vi "fita2.vi"() -> ()   [LabVIEW 2014]
uses:
  <vilib>/Analysis/5stat.llb/RMS (DBL).vi
  <vilib>/DAQmx/create/channels.llb/DAQmx Create Channel (AI-Voltage-Basic).vi
  <vilib>/DAQmx/configure/timing.llb/DAQmx Timing (Sample Clock).vi
  <vilib>/DAQmx/read.llb/DAQmx Read (Analog 1D Wfm NChan NSamp).vi
  <vilib>/Waveform/WDTOps.llb/WDT Index Channel DBL.vi
  <vilib>/Utility/file.llb/Write To Spreadsheet File (string).vi
  <vilib>/Analysis/NI_AALPro.lvlib
panel:
  out "CH4":dbl
  out "CH3":dbl
  out "CH2":dbl
  out "CH1":dbl
  out "MIN CH4":bool
  out "MIN CH2":bool
  out "MIN CH1":bool
  out "MIN CH3":bool
  out "MAX CH4":bool
  out "MAX CH3":bool
  out "MAX CH2":bool
  out "MAX CH1":bool
  in  "Temp Max CH2":dbl
  in  "Temp Min CH1":dbl
  in  "Temp Min CH2":dbl
  in  "Temp Max CH3":dbl
  in  "Temp Min CH3":dbl
  in  "Temp Max CH4":dbl
  in  "Temp Min CH4":dbl
  in  "Temp Max CH1":dbl
  in  "Start":bool
  in  "stop":bool
  out "Waveform Chart":T1(graph)
  out "Canals seleccionats":dbl
  in  "Durada adquisicio":dbl
  in  "Temps entre adquisicio":dbl
  in  "Numero de mostres per fer mitja":u32
  in  "Nombre de Canals":string(combo)
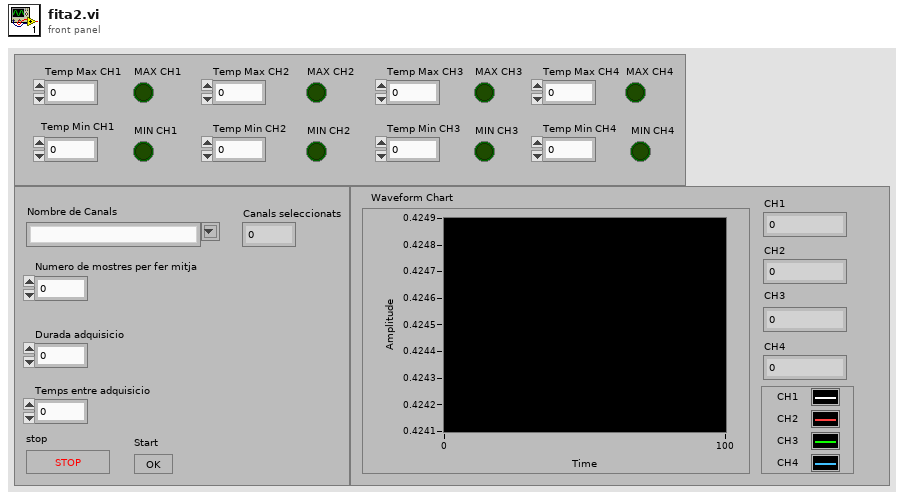
[diagram p1: front panel]
types:
  T1 = cluster{"rms value":dbl, "rms value":dbl, "rms value":dbl, "rms value":dbl}
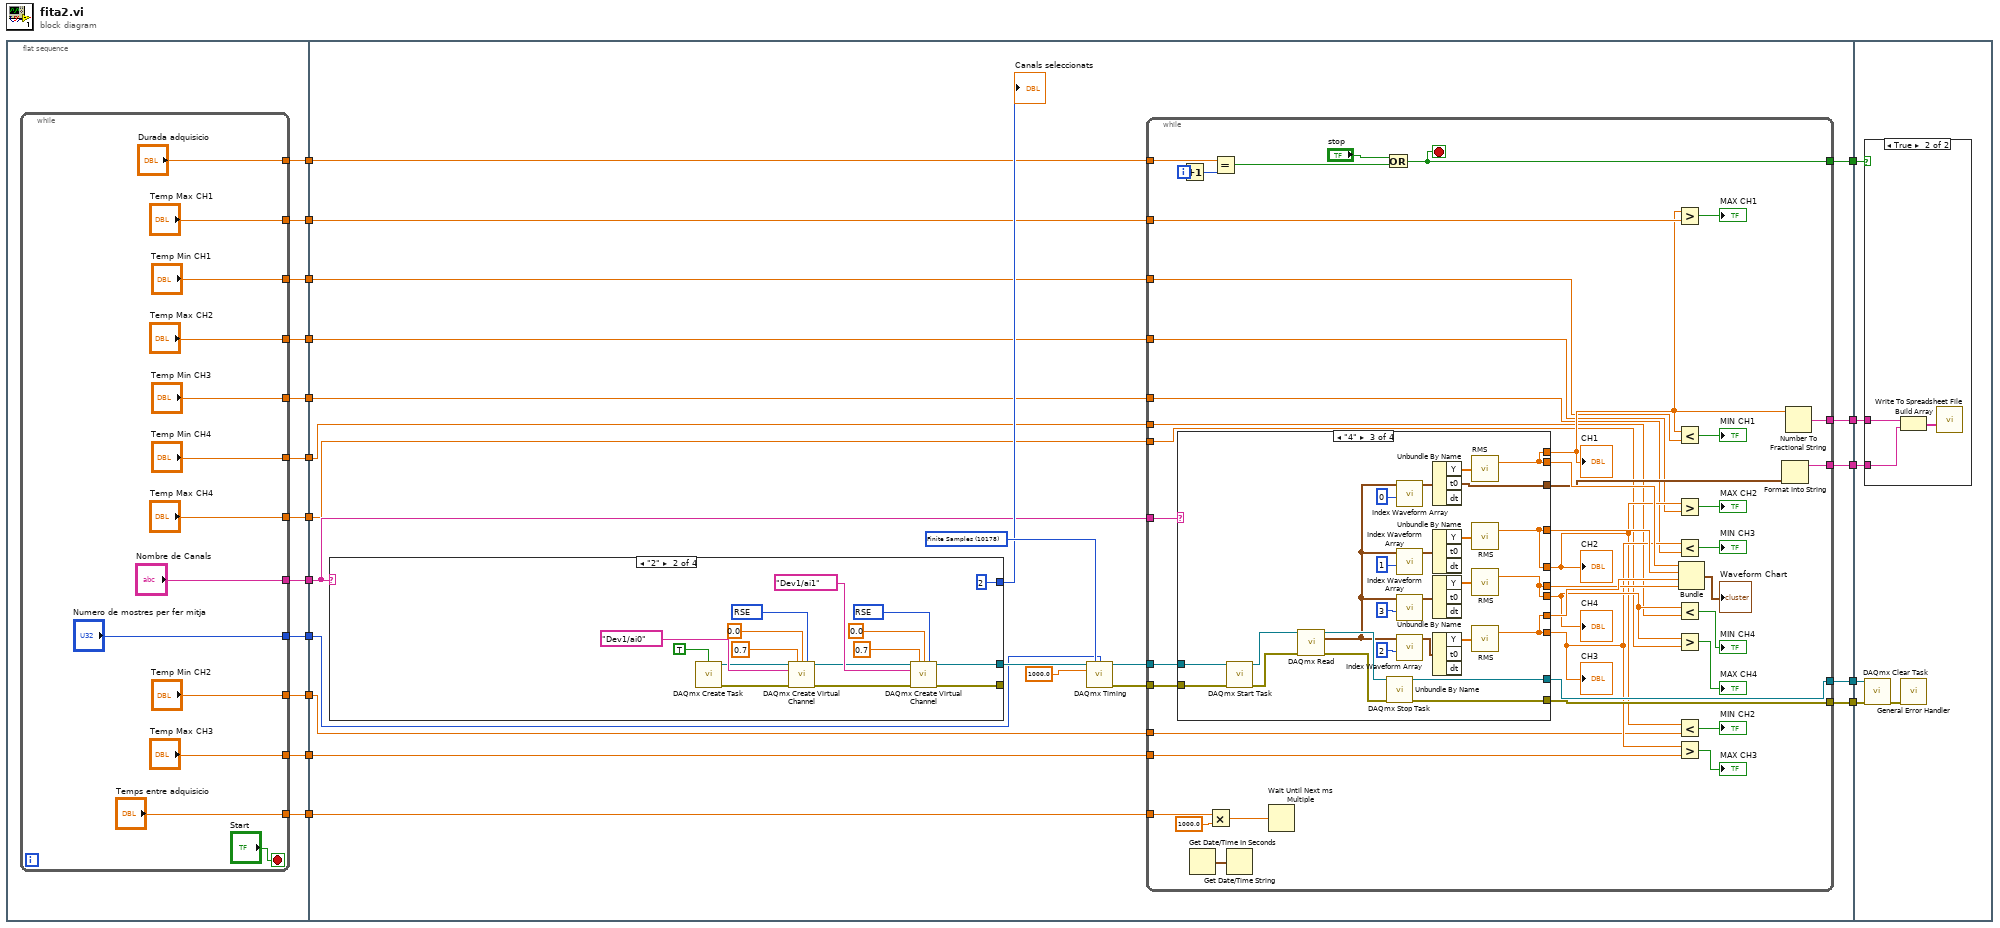
[diagram p0: block diagram]
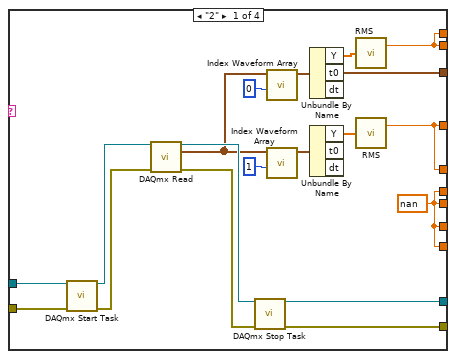
[diagram p2: hidden frame]
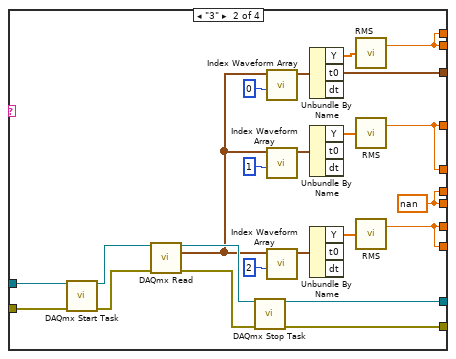
[diagram p3: hidden frame]
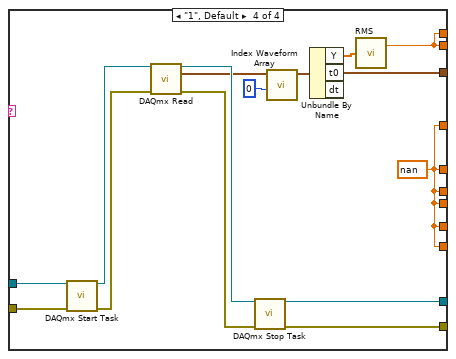
[diagram p4: hidden frame]
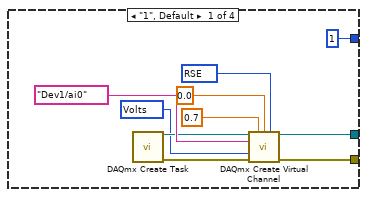
[diagram p5: hidden frame]
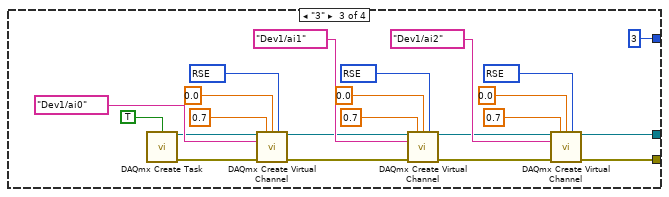
[diagram p6: hidden frame]
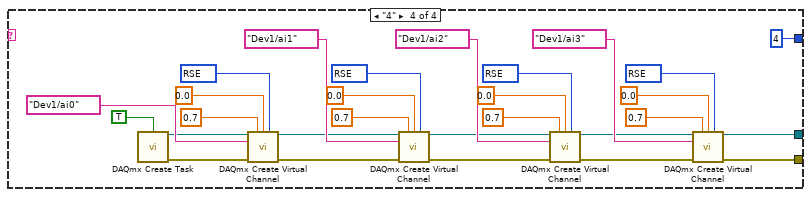
[diagram p7: hidden frame]
diagram:
  n1 = flat-sequence {
    tunnel: [w29] -> w17
    tunnel: [w28] -> w16
    tunnel: [w27] -> w15
    tunnel: [w26] -> w14
    tunnel: [w25] -> w8
    tunnel: [w24] -> w7
    tunnel: [w23] -> w6
    tunnel: [w22] -> w5
    tunnel: [w21] -> w4
    tunnel: [w20] -> w3
    tunnel: [w19] -> w2
    tunnel: [w18] -> w1
    tunnel: w17 -> [w59]
    tunnel: w16 -> [w58]
    tunnel: w15 -> [w57]
    tunnel: w14 -> [w56]
    tunnel: [w55] -> w13
    tunnel: [w54] -> w12
    tunnel: [w53] -> w11
    tunnel: [w52] -> w10
    tunnel: [w51] -> w9
    tunnel: w8 -> [w50]
    tunnel: w7 -> [w49]
    tunnel: w6 -> [w48]
    tunnel: w5 -> [w47]
    tunnel: w4 -> [w46]
    tunnel: w3 -> [w45]
    tunnel: w2 -> [w44]
    tunnel: w1 -> [w43]
    tunnel: w13 -> [w272]
    tunnel: w12 -> [w271]
    tunnel: w11 -> [w270]
    tunnel: w10 -> [w269]
    tunnel: w9 -> [w268]
    frame #0 {
      n2 = while {
        tunnel: ["Nombre de Canals"] -> w29
        tunnel: ["Durada adquisicio"] -> w28
        tunnel: ["Temps entre adquisicio"] -> w27
        tunnel: ["Numero de mostres per fer mitja"] -> w26
        tunnel: ["Temp Max CH1"] -> w25
        tunnel: ["Temp Min CH1"] -> w24
        tunnel: ["Temp Max CH3"] -> w23
        tunnel: ["Temp Max CH2"] -> w22
        tunnel: ["Temp Max CH4"] -> w21
        tunnel: ["Temp Min CH3"] -> w20
        tunnel: ["Temp Min CH2"] -> w19
        tunnel: ["Temp Min CH4"] -> w18
        stop <- "Start" stop-if-true
      }
    }
    frame #1 {
      w64 = 10178 items=["Finite Samples"=10178, "Continuous Samples"=10123, "Hardware Timed Single Point"=12522] ("sample mode")
      n3 = case shown="\"2\"" w59 {
        tunnel: [w195 w204 w220 w242] -> w65
        tunnel: [w194 w203 w219 w241] -> _
        tunnel: [1 2 3 4] -> w63
        frame "1", Default {
          w192 = 10348 items=["Volts"=10348, "From Custom Scale"=10065] ("units")
          w198 = 10083 items=["default"=-1, "RSE"=10083, "NRSE"=10078, "Differential"=10106, "Pseudodifferential"=12529] ("input terminal configuration")
          n4 = call <vilib>:"DAQmx Create Task.vi"() -> ("task out"=w196:refnum<k21>, "error out"=w197:errorcluster)  [unwired: 14 in]
          n5 = call-poly <vilib>:"DAQmx Create Virtual Channel.vi"("task in"=w196, "maximum value"=0.7, "minimum value"=0.0, "input terminal configuration"=w198, "physical channels"=tag "Dev1/ai0", "units"=w192, "error in"=w197) -> ("task out"=w195:refnum<k21>, "error out"=w194:errorcluster)  [unwired: 7 in]
        }
        frame "2" {
          w207 = 10083 items=["default"=-1, "RSE"=10083, "NRSE"=10078, "Differential"=10106, "Pseudodifferential"=12529] ("input terminal configuration")
          w214 = 10083 items=["default"=-1, "RSE"=10083, "NRSE"=10078, "Differential"=10106, "Pseudodifferential"=12529] ("input terminal configuration")
          n6 = call <vilib>:"DAQmx Create Task.vi"("auto cleanup"=TRUE) -> ("task out"=w212:refnum<k21>, "error out"=w213:errorcluster)  [unwired: 13 in]
          n7 = call-poly <vilib>:"DAQmx Create Virtual Channel.vi"("task in"=w212, "maximum value"=0.7, "minimum value"=0.0, "input terminal configuration"=w214, "physical channels"=tag "Dev1/ai0", "error in"=w213) -> ("task out"=w206:refnum<k21>, "error out"=w205:errorcluster)  [unwired: 8 in]
          n8 = call-poly <vilib>:"DAQmx Create Virtual Channel.vi"("task in"=w206, "maximum value"=0.7, "minimum value"=0.0, "input terminal configuration"=w207, "physical channels"=tag "Dev1/ai1", "error in"=w205) -> ("task out"=w204:refnum<k21>, "error out"=w203:errorcluster)  [unwired: 8 in]
        }
        frame "3" {
          w223 = 10083 items=["default"=-1, "RSE"=10083, "NRSE"=10078, "Differential"=10106, "Pseudodifferential"=12529] ("input terminal configuration")
          w229 = 10083 items=["default"=-1, "RSE"=10083, "NRSE"=10078, "Differential"=10106, "Pseudodifferential"=12529] ("input terminal configuration")
          w236 = 10083 items=["default"=-1, "RSE"=10083, "NRSE"=10078, "Differential"=10106, "Pseudodifferential"=12529] ("input terminal configuration")
          n9 = call <vilib>:"DAQmx Create Task.vi"("auto cleanup"=TRUE) -> ("task out"=w234:refnum<k21>, "error out"=w235:errorcluster)  [unwired: 13 in]
          n10 = call-poly <vilib>:"DAQmx Create Virtual Channel.vi"("task in"=w234, "maximum value"=0.7, "minimum value"=0.0, "input terminal configuration"=w236, "physical channels"=tag "Dev1/ai0", "error in"=w235) -> ("task out"=w228:refnum<k21>, "error out"=w227:errorcluster)  [unwired: 8 in]
          n11 = call-poly <vilib>:"DAQmx Create Virtual Channel.vi"("task in"=w228, "maximum value"=0.7, "minimum value"=0.0, "input terminal configuration"=w229, "physical channels"=tag "Dev1/ai1", "error in"=w227) -> ("task out"=w222:refnum<k21>, "error out"=w221:errorcluster)  [unwired: 8 in]
          n12 = call-poly <vilib>:"DAQmx Create Virtual Channel.vi"("task in"=w222, "maximum value"=0.7, "minimum value"=0.0, "input terminal configuration"=w223, "physical channels"=tag "Dev1/ai2", "error in"=w221) -> ("task out"=w220:refnum<k21>, "error out"=w219:errorcluster)  [unwired: 8 in]
        }
        frame "4" {
          w245 = 10083 items=["default"=-1, "RSE"=10083, "NRSE"=10078, "Differential"=10106, "Pseudodifferential"=12529] ("input terminal configuration")
          w251 = 10083 items=["default"=-1, "RSE"=10083, "NRSE"=10078, "Differential"=10106, "Pseudodifferential"=12529] ("input terminal configuration")
          w257 = 10083 items=["default"=-1, "RSE"=10083, "NRSE"=10078, "Differential"=10106, "Pseudodifferential"=12529] ("input terminal configuration")
          w264 = 10083 items=["default"=-1, "RSE"=10083, "NRSE"=10078, "Differential"=10106, "Pseudodifferential"=12529] ("input terminal configuration")
          n13 = call <vilib>:"DAQmx Create Task.vi"("auto cleanup"=TRUE) -> ("task out"=w262:refnum<k21>, "error out"=w263:errorcluster)  [unwired: 13 in]
          n14 = call-poly <vilib>:"DAQmx Create Virtual Channel.vi"("task in"=w262, "maximum value"=0.7, "minimum value"=0.0, "input terminal configuration"=w264, "physical channels"=tag "Dev1/ai0", "error in"=w263) -> ("task out"=w256:refnum<k21>, "error out"=w255:errorcluster)  [unwired: 8 in]
          n15 = call-poly <vilib>:"DAQmx Create Virtual Channel.vi"("task in"=w256, "maximum value"=0.7, "minimum value"=0.0, "input terminal configuration"=w257, "physical channels"=tag "Dev1/ai1", "error in"=w255) -> ("task out"=w250:refnum<k21>, "error out"=w249:errorcluster)  [unwired: 8 in]
          n16 = call-poly <vilib>:"DAQmx Create Virtual Channel.vi"("task in"=w250, "maximum value"=0.7, "minimum value"=0.0, "input terminal configuration"=w251, "physical channels"=tag "Dev1/ai2", "error in"=w249) -> ("task out"=w244:refnum<k21>, "error out"=w243:errorcluster)  [unwired: 8 in]
          n17 = call-poly <vilib>:"DAQmx Create Virtual Channel.vi"("task in"=w244, "maximum value"=0.7, "minimum value"=0.0, "input terminal configuration"=w245, "physical channels"=tag "Dev1/ai3", "error in"=w243) -> ("task out"=w242:refnum<k21>, "error out"=w241:errorcluster)  [unwired: 8 in]
        }
      }
      "Canals seleccionats" <- w63
      n18 = call-poly <vilib>:"DAQmx Timing.vi"("task/channels in"=w65, "sample mode"=w64, "samples per channel"=w56, "rate"=1000.0) -> ("task out"=w61:refnum<k21>, "error out"=w60:errorcluster)  [unwired: 10 in]
      n19 = while {
        tunnel: w57 -> [w106]
        tunnel: w59 -> [w105]
        tunnel: w61 -> [w104]
        tunnel: w60 -> [w103]
        tunnel: [w102] -> w55
        tunnel: [w101] -> w54
        tunnel: w58 -> [w92]
        tunnel: [w91] -> w53
        tunnel: [w87] -> w52
        tunnel: [w88] -> w51
        tunnel: w50 -> [w86]
        tunnel: w49 -> [w82]
        tunnel: w48 -> [w71]
        tunnel: w47 -> [w70]
        tunnel: w46 -> [w69]
        tunnel: w45 -> [w68]
        tunnel: w44 -> [w67]
        tunnel: w43 -> [w66]
        i -> [w98]
        stop <- w91 stop-if-true
        n20 = case shown="\"4\"" w105 {
          tunnel: w104 -> [w116 w136 w159 w183]
          tunnel: w103 -> [w115 w135 w158 w182]
          tunnel: [w114 w134 w157 w181] -> w102
          tunnel: [w113 w133 w156 w180] -> w101
          tunnel: [w112 w131 w155 w179] -> w96
          tunnel: [w111 w130 w154 w178] -> w95
          tunnel: [w110 w132 w153 w178] -> w93
          tunnel: [w110 w129 w152 w178] -> w75
          tunnel: [w112 w131 w155 w179] -> w85
          tunnel: [w111 w130 w154 w178] -> w72
          tunnel: [w110 w132 w153 w178] -> w73
          tunnel: [w110 w129 w152 w178] -> w74
          tunnel: [w109 w128 w151 w177] -> w89
          frame "2" {
            w110 = nan ("rms value")
            n21 = call <vilib>:"DAQmx Start Task.vi"("task/channels in"=w116, "error in"=w115) -> ("task out"=w127:refnum<k21>, "error out"=w126:errorcluster)  [unwired: 12 in]
            n22 = call-poly <vilib>:"DAQmx Read.vi"("task/channels in"=w127, "error in"=w126) -> ("task out"=w124:refnum<k21>, "data"=w117:waveform(dbl)[], "error out"=w125:errorcluster)  [unwired: 11 in]
            n23 = call <vilib>:"DAQmx Stop Task.vi"("task/channels in"=w124, "error in"=w125) -> ("task out"=w114:refnum<k21>, "error out"=w113:errorcluster)  [unwired: 12 in]
            n24 = call-poly <vilib>:"Index Waveform Array.vi"("index"=0, "waveform array"=w117) -> ("waveform"=w119:waveform(dbl))  [unwired: 8 in, 1 out]
            n25 = call-poly <vilib>:"Index Waveform Array.vi"("index"=1, "waveform array"=w117) -> ("waveform"=w122:waveform(dbl))  [unwired: 8 in, 1 out]
            n26 = Unbundle By Name(w119) -> ("Y"=w118:dbl[], "t0"=w109:timestamp)  [unwired: 1 out]
            n27 = Unbundle By Name(w122) -> ("Y"=w121:dbl[])  [unwired: 2 out]
            n28 = call-poly <vilib>:"RMS.vi"("X"=w118) -> ("rms value"=w112:dbl)  [unwired: 1 out]
            n29 = call-poly <vilib>:"RMS.vi"("X"=w121) -> ("rms value"=w111:dbl)  [unwired: 1 out]
          }
          frame "3" {
            w129 = nan ("rms value")
            n30 = call <vilib>:"DAQmx Start Task.vi"("task/channels in"=w136, "error in"=w135) -> ("task out"=w150:refnum<k21>, "error out"=w149:errorcluster)  [unwired: 12 in]
            n31 = call-poly <vilib>:"DAQmx Read.vi"("task/channels in"=w150, "error in"=w149) -> ("task out"=w147:refnum<k21>, "data"=w137:waveform(dbl)[], "error out"=w148:errorcluster)  [unwired: 11 in]
            n32 = call <vilib>:"DAQmx Stop Task.vi"("task/channels in"=w147, "error in"=w148) -> ("task out"=w134:refnum<k21>, "error out"=w133:errorcluster)  [unwired: 12 in]
            n33 = call-poly <vilib>:"Index Waveform Array.vi"("index"=0, "waveform array"=w137) -> ("waveform"=w142:waveform(dbl))  [unwired: 8 in, 1 out]
            n34 = call-poly <vilib>:"Index Waveform Array.vi"("index"=1, "waveform array"=w137) -> ("waveform"=w139:waveform(dbl))  [unwired: 8 in, 1 out]
            n35 = call-poly <vilib>:"Index Waveform Array.vi"("index"=2, "waveform array"=w137) -> ("waveform"=w145:waveform(dbl))  [unwired: 8 in, 1 out]
            n36 = Unbundle By Name(w142) -> ("Y"=w141:dbl[], "t0"=w128:timestamp)  [unwired: 1 out]
            n37 = Unbundle By Name(w139) -> ("Y"=w138:dbl[])  [unwired: 2 out]
            n38 = Unbundle By Name(w145) -> ("Y"=w144:dbl[])  [unwired: 2 out]
            n39 = call-poly <vilib>:"RMS.vi"("X"=w141) -> ("rms value"=w131:dbl)  [unwired: 1 out]
            n40 = call-poly <vilib>:"RMS.vi"("X"=w138) -> ("rms value"=w130:dbl)  [unwired: 1 out]
            n41 = call-poly <vilib>:"RMS.vi"("X"=w144) -> ("rms value"=w132:dbl)  [unwired: 1 out]
          }
          frame "4" {
            n42 = call <vilib>:"DAQmx Start Task.vi"("task/channels in"=w159, "error in"=w158) -> ("task out"=w176:refnum<k21>, "error out"=w175:errorcluster)  [unwired: 12 in]
            n43 = call-poly <vilib>:"DAQmx Read.vi"("task/channels in"=w176, "error in"=w175) -> ("task out"=w173:refnum<k21>, "data"=w160:waveform(dbl)[], "error out"=w174:errorcluster)  [unwired: 11 in]
            n44 = call <vilib>:"DAQmx Stop Task.vi"("task/channels in"=w173, "error in"=w174) -> ("task out"=w157:refnum<k21>, "error out"=w156:errorcluster)  [unwired: 12 in]
            n45 = call-poly <vilib>:"Index Waveform Array.vi"("index"=0, "waveform array"=w160) -> ("waveform"=w165:waveform(dbl))  [unwired: 8 in, 1 out]
            n46 = call-poly <vilib>:"Index Waveform Array.vi"("index"=1, "waveform array"=w160) -> ("waveform"=w162:waveform(dbl))  [unwired: 8 in, 1 out]
            n47 = call-poly <vilib>:"Index Waveform Array.vi"("index"=3, "waveform array"=w160) -> ("waveform"=w168:waveform(dbl))  [unwired: 8 in, 1 out]
            n48 = call-poly <vilib>:"Index Waveform Array.vi"("index"=2, "waveform array"=w160) -> ("waveform"=w171:waveform(dbl))  [unwired: 8 in, 1 out]
            n49 = Unbundle By Name(w165) -> ("Y"=w164:dbl[], "t0"=w151:timestamp)  [unwired: 1 out]
            n50 = Unbundle By Name(w162) -> ("Y"=w161:dbl[])  [unwired: 2 out]
            n51 = Unbundle By Name(w168) -> ("Y"=w167:dbl[])  [unwired: 2 out]
            n52 = Unbundle By Name(w171) -> ("Y"=w170:dbl[])  [unwired: 2 out]
            n53 = call-poly <vilib>:"RMS.vi"("X"=w164) -> ("rms value"=w155:dbl)  [unwired: 1 out]
            n54 = call-poly <vilib>:"RMS.vi"("X"=w161) -> ("rms value"=w154:dbl)  [unwired: 1 out]
            n55 = call-poly <vilib>:"RMS.vi"("X"=w167) -> ("rms value"=w152:dbl)  [unwired: 1 out]
            n56 = call-poly <vilib>:"RMS.vi"("X"=w170) -> ("rms value"=w153:dbl)  [unwired: 1 out]
          }
          frame "1", Default {
            w178 = nan ("rms value")
            n57 = call <vilib>:"DAQmx Start Task.vi"("task/channels in"=w183, "error in"=w182) -> ("task out"=w191:refnum<k21>, "error out"=w190:errorcluster)  [unwired: 12 in]
            n58 = call-poly <vilib>:"DAQmx Read.vi"("task/channels in"=w191, "error in"=w190) -> ("task out"=w188:refnum<k21>, "data"=w184:waveform(dbl)[], "error out"=w189:errorcluster)  [unwired: 11 in]
            n59 = call <vilib>:"DAQmx Stop Task.vi"("task/channels in"=w188, "error in"=w189) -> ("task out"=w181:refnum<k21>, "error out"=w180:errorcluster)  [unwired: 12 in]
            n60 = call-poly <vilib>:"Index Waveform Array.vi"("index"=0, "waveform array"=w184) -> ("waveform"=w186:waveform(dbl))  [unwired: 8 in, 1 out]
            n61 = Unbundle By Name(w186) -> ("Y"=w185:dbl[], "t0"=w177:timestamp)  [unwired: 1 out]
            n62 = call-poly <vilib>:"RMS.vi"("X"=w185) -> ("rms value"=w179:dbl)  [unwired: 1 out]
          }
        }
        "CH1" <- w85
        "CH2" <- w72
        "CH3" <- w73
        "CH4" <- w74
        n63 = Increment(x=w98) -> (x+1=w97:i32)
        n64 = Get Date/Time In Seconds() -> (seconds since 1Jan1904=w90:timestamp)
        n65 = Multiply(x=w106, y=1000.0) -> (x*y=w107:dbl)
        n66 = Equal?(x=w92, y=w97) -> (x = y?=w99:bool)
        n67 = Get Date/Time String(seconds (now)=w90) -> ()  [unwired: 2 in, 2 out]
        n68 = Wait Until Next ms Multiple(millisecond multiple=w107) -> ()  [unwired: 1 out]
        n69 = Or(x="stop", y=w99) -> (x .or. y?=w91:bool)
        n70 = Greater?(x=w85, y=w86) -> (0:→"MAX CH1":bool)
        n71 = Less?(x=w85, y=w82) -> (x < y?=→"MIN CH1":bool)
        n72 = Greater?(x=w72, y=w70) -> (0:→"MAX CH2":bool)
        n73 = Less?(x=w73, y=w68) -> (x < y?=→"MIN CH3":bool)
        n74 = Less?(x=w74, y=w66) -> (x < y?=→"MIN CH4":bool)
        n75 = Greater?(x=w74, y=w69) -> (0:→"MAX CH4":bool)
        n76 = Less?(x=w72, y=w67) -> (x < y?=→"MIN CH2":bool)
        n77 = Greater?(x=w73, y=w71) -> (0:→"MAX CH3":bool)
        n78 = Bundle("rms value"=w96, "rms value"=w95, "rms value"=w93, "rms value"=w75) -> (→"Waveform Chart":T1)  [unwired: 1 in]
        n79 = Format Into String(w89) -> (resulting string=w88:string)  [unwired: 3 in, 1 out]
        n80 = Number To Fractional String(number=w85) -> (F-format string=w87:string)  [unwired: 3 in]
      }
    }
    frame #2 {
      n81 = case shown="True" w270 {
        tunnel: w269 -> [_ w276]
        tunnel: w268 -> [_ w275]
        frame False {
        }
        frame True {
          n82 = Build Array(w276, w275) -> (w274:string[])
          n83 = call-poly <vilib>:"Write To Spreadsheet File.vi"("1D data"=w274) -> ()  [unwired: 7 in, 1 out]
        }
      }
      n84 = call <vilib>:"DAQmx Clear Task.vi"("task in"=w272, "error in"=w271) -> ("error out"=w273:errorcluster)  [unwired: 13 in]
      n85 = call <vilib>:"General Error Handler.vi"("error in (no error)"=w273) -> ()  [unwired: 10 in, 5 out]
    }
  }
